vi "总磷总氮测量数据储存.vi"   [LabVIEW 2016, in "斯坦道总氮V2.lvlib"]
uses:
  <vilib>/ptbypt/NI_PtbyPt.lvlib
types:
  T1 = cluster{"跨度值":dbl, "零点标准液浓度":dbl, "跨度标准液浓度":dbl, "标准液标准浓度":dbl}
  T2 = cluster{"系统时间":timestamp, "工作状态":u16, "测量模式":enum16{"待机", "连续模式", "周期模式", "定点模式", "受控模式", "手动模式"}, "告警代码":u16, "故障代码":u16, "日志代码":u16, "软件版本":u16, "F0":sgl, "F1":sgl, "F2":sgl, "F3":sgl, "T":sgl, "H":sgl, "id":u16, "flowid":u16, "量程":u16, "总磷控温温度1":sgl, "营养盐控温温度2":sgl, "ADC":sgl}
  T3 = cluster{"运行模式":enum16{"维护模式", "常规模式", "应急模式", "质控模式", "性能测试"}, "质控频次":enum16{"关闭", "每天", "星期一", "星期二", "星期三", "星期四", "星期五", "星期六", "星期日"}, "空白核查时间":u16, "跨度核查时间":u16, "测量间隔":dbl}
  T4 = cluster{"因子编码":u32, "单位":u16, "标样参考值":sgl, "水样数据时间":timestamp, "水样实测值":sgl, "水样数据标识":string, "标样数据时间":timestamp, "标样实测值":sgl, "标样数据标识":string, "空白数据时间":timestamp, "空白实测值":sgl, "空白数据标识":string, "零点核查数据时间":timestamp, "零点核查实测值":sgl, "零点核查数据标识":string, "跨度核查数据时间":timestamp, "跨度核查实测值":sgl, "跨度核查数据标识":string, "加标回收数据时间":timestamp, "加标回收实测值":sgl, "加标回收数据标识":string, "平行样数据时间":timestamp, "平行样实测值":sgl, "平行样数据标识":string, "F0":sgl, "F1":sgl, "F2":sgl, "F3":sgl, "F4":sgl, "F5":sgl, "F6":sgl, "F7":sgl, "温度":sgl, "湿度":sgl, "X值":sgl, "fidrange":u16}[]
  T5 = cluster{"系统时间":timestamp, "工作状态":u16, "测量模式":enum16{"待机", "连续模式", "周期模式", "定点模式", "受控模式", "手动模式"}, "告警代码":u16, "故障代码":u16, "日志代码":u16, "软件版本":u16, "F0":sgl, "F1":sgl, "F2":sgl, "F3":sgl, "T":sgl, "H":sgl, "id":u16, "flowid":u16, "量程":u16, "总磷控温温度1":sgl, "营养盐控温温度2":sgl, "ADC":sgl}[]
  T6 = cluster{"总磷跨度值":dbl, "总磷零点标准液浓度":dbl, "总磷跨度标准液浓度":dbl, "总磷标准液标准浓度":dbl, "总氮跨度值":dbl, "总氮零点标准液浓度":dbl, "总氮跨度标准液浓度":dbl, "总氮标准液标准浓度":dbl, "氨氮跨度值":dbl, "氨氮零点标准液浓度":dbl, "氨氮跨度标准液浓度":dbl, "氨氮标准液标准浓度":dbl}
  T7 = cluster{"因子编码":u32, "单位":u16, "标样参考值":sgl, "水样数据时间":timestamp, "水样实测值":sgl, "水样数据标识":string, "标样数据时间":timestamp, "标样实测值":sgl, "标样数据标识":string, "空白数据时间":timestamp, "空白实测值":sgl, "空白数据标识":string, "零点核查数据时间":timestamp, "零点核查实测值":sgl, "零点核查数据标识":string, "跨度核查数据时间":timestamp, "跨度核查实测值":sgl, "跨度核查数据标识":string, "加标回收数据时间":timestamp, "加标回收实测值":sgl, "加标回收数据标识":string, "平行样数据时间":timestamp, "平行样实测值":sgl, "平行样数据标识":string, "F0":sgl, "F1":sgl, "F2":sgl, "F3":sgl, "F4":sgl, "F5":sgl, "F6":sgl, "F7":sgl, "温度":sgl, "湿度":sgl, "X值":sgl, "fidrange":u16}
  T8 = cluster{"时间标识":timestamp, "测量模式":enum16{"维护数据", "水样测试", "标样核查", "零点核查", "跨度核查", "空白测试", "平行样测试", "加标回收", "空白校准", "标样校准", "初始化（清洗）", "快捷测试"}, "数据标记表":string, "监测值":sgl, "单位":u16, "数据标识":string, "因子编码":u32, "标样参考值":sgl, "F0":sgl, "F1":sgl, "F2":sgl, "F3":sgl, "F4":sgl, "F5":sgl, "F6":sgl, "F7":sgl, "X":sgl, "温度":sgl, "湿度":sgl, "量程标识":string, "SN":string, "跨度值":sgl, "X1":sgl}
  T9 = typedef "斯坦道总氮V2.lvlib/关键参数.ctl" = cluster{"测量量程":sgl, "测量检出限":sgl, "测量精度":sgl, "测量间隔":sgl, "消解温度":sgl, "消解时长":sgl, "三项式系数":sgl, "二次多项式系数":sgl, "曲线斜率":sgl, "曲线截距":sgl, "线性相关系数":sgl, "空白校准时间":timestamp, "标样校准时间":timestamp, "测量信号值":sgl, "稀释倍数":sgl, "空白标定系数":sgl, "量程系数":sgl}
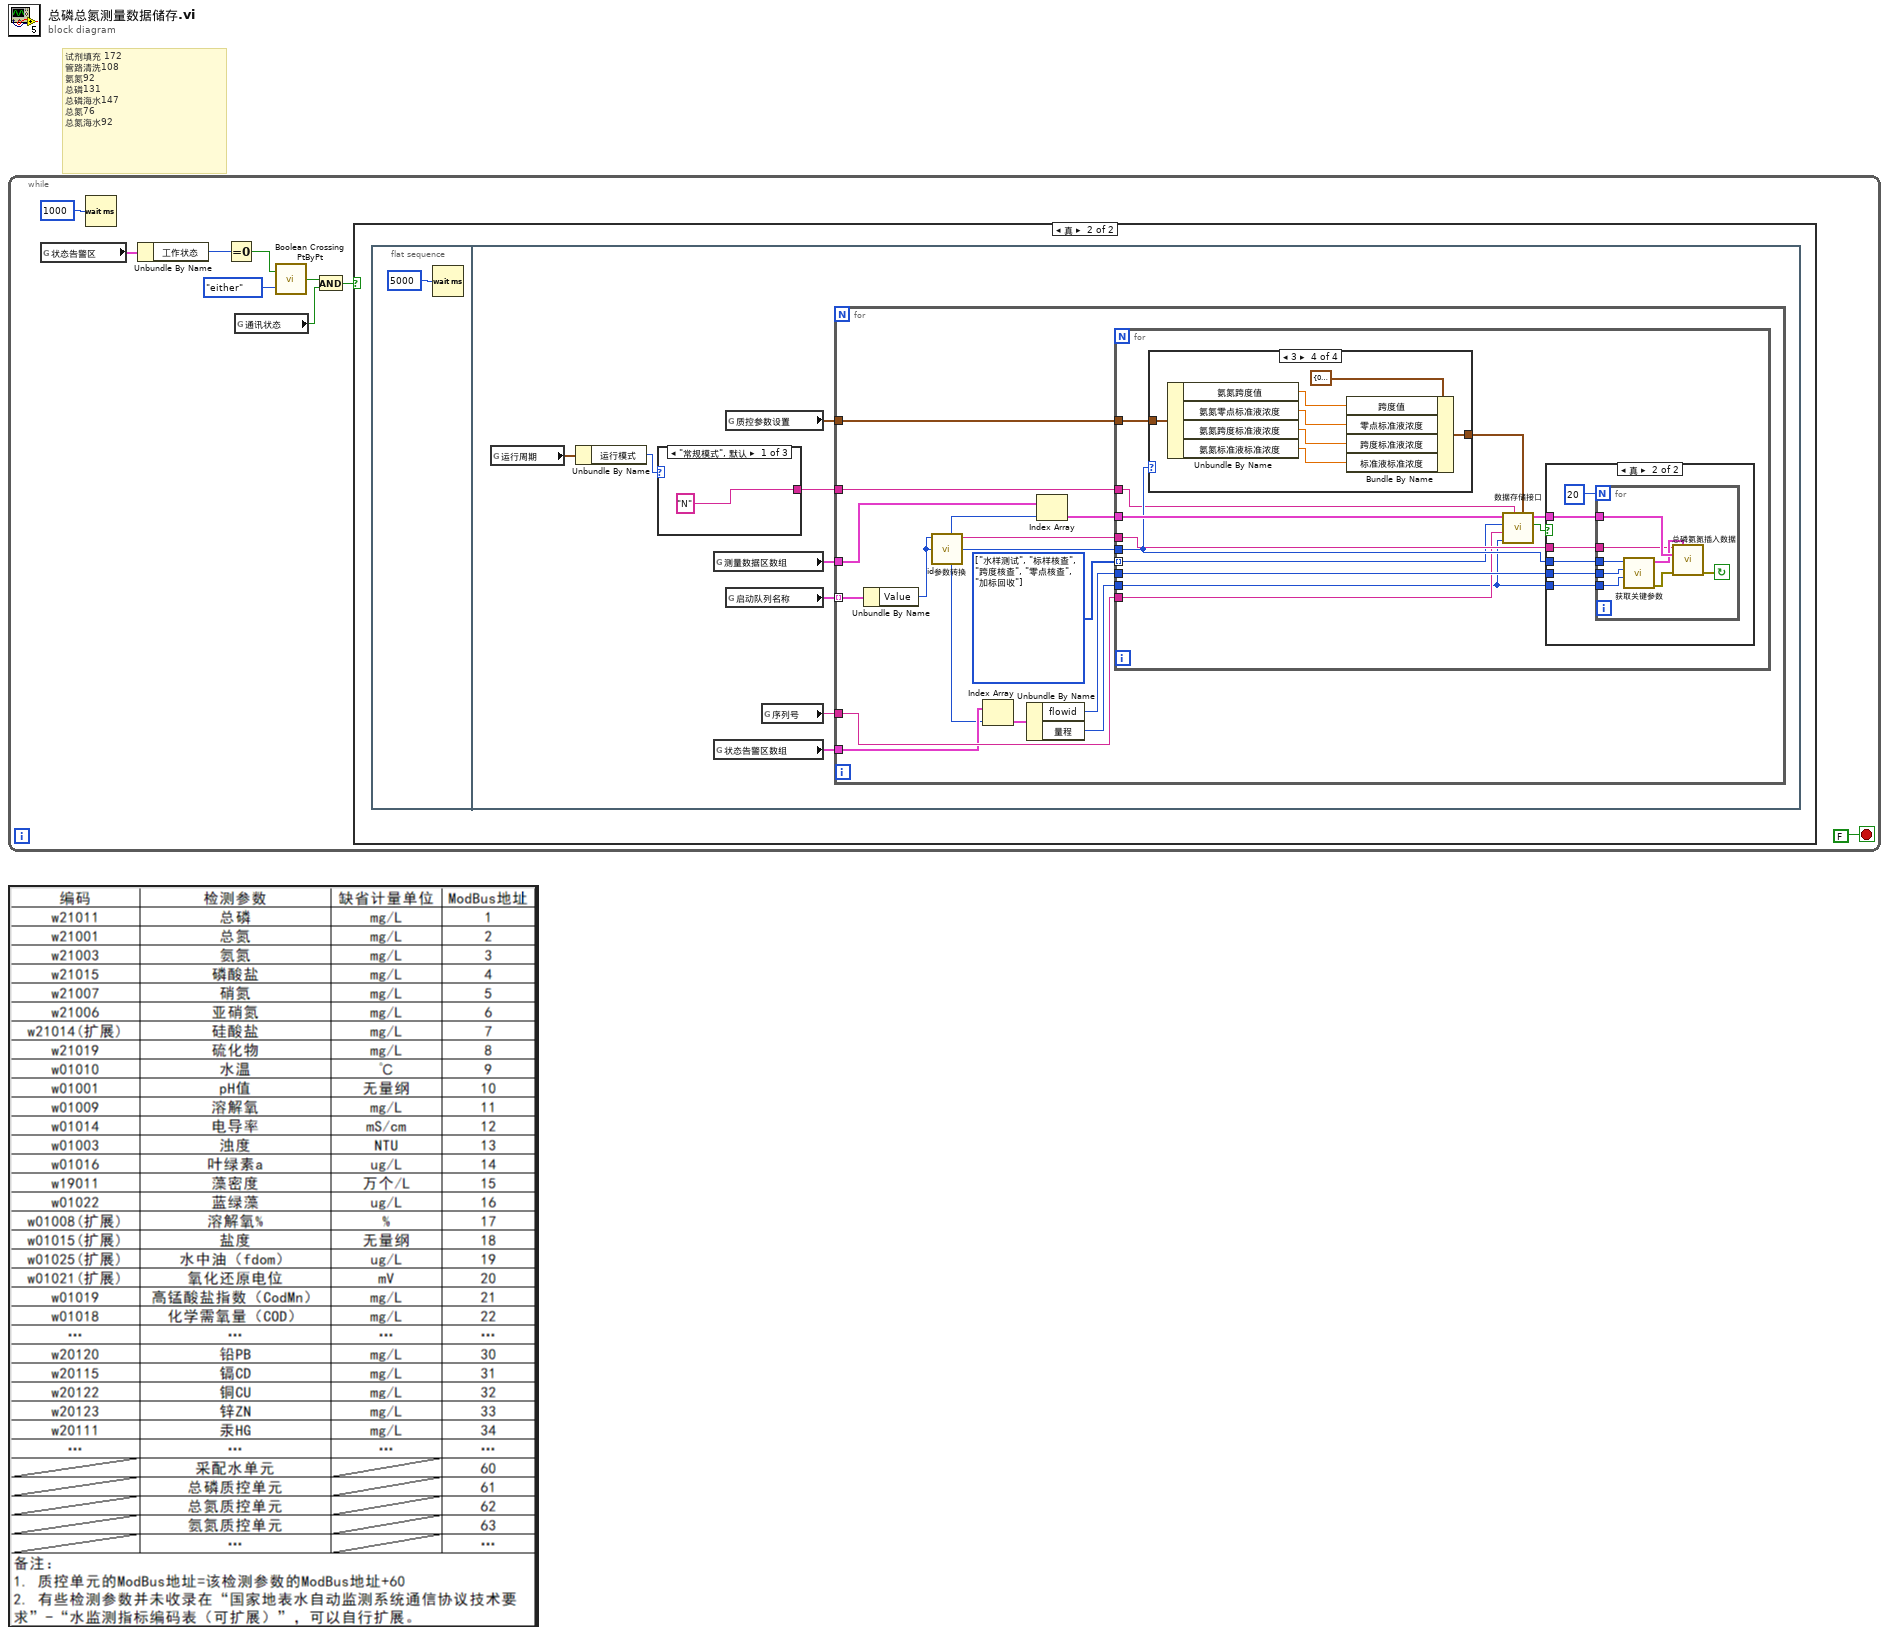
[diagram p0: block diagram]
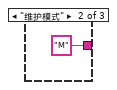
[diagram p3: hidden frame]
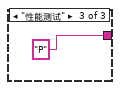
[diagram p4: hidden frame]
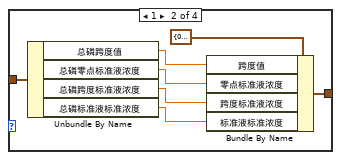
[diagram p7: hidden frame]
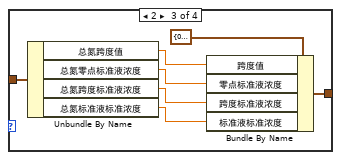
[diagram p8: hidden frame]
diagram:
  # "试剂填充 172 \n管路清洗108\n氨氮92\n总磷131\n总磷海水147\n总氮76\n总氮海水92"
  n1 = while {
    stop <- FALSE stop-if-true
    n2 = global read "VAR总磷总氮全局变量.vi" "状态告警区"() -> (w8:T2)
    n3 = Wait (ms)(milliseconds to wait=u32 1000 ("等待时间（毫秒）")) -> ()  [unwired: 1 out]
    n4 = Unbundle By Name(w8) -> ("工作状态"=w6:u16)
    n5 = Equal To 0?(x=w6) -> (x = 0?=w3:bool)
    n6 = global read "VAR总磷总氮全局变量.vi" "通讯状态"() -> (w1:bool)
    n7 = call <vilib>:"Boolean Crossing PtByPt.vi"("direction"=enum16{"either", "false-true", "true-false"}."either", "input"=w3) -> ("crossing"=w4:bool)  [unwired: 1 in]
    n8 = And(x=w4, y=w1) -> (x .and. y?=w2:bool)
    n9 = case shown="真" w2 {
      frame False {
      }
      frame True {
        n10 = flat-sequence {
          frame #0 {
            n11 = Wait (ms)(milliseconds to wait=u32 5000 ("等待时间（毫秒）")) -> ()  [unwired: 1 out]
          }
          frame #1 {
            n12 = global read "总磷总氮断电保存全局变量.vi" "运行周期"() -> (w14:T3)
            n13 = Unbundle By Name(w14) -> ("运行模式"=w12:enum16{"维护模式", "常规模式", "应急模式", "质控模式", "性能测试"})
            n14 = case shown="\"常规模式\", 默认" w12 {
              tunnel: ["N" "M" "P"] -> w11
              frame "常规模式", Default {
              }
              frame "维护模式" {
              }
              frame "性能测试" {
              }
            }
            n15 = global read "VAR总磷总氮全局变量.vi" "测量数据区数组"() -> (w15:T4)
            n16 = global read "VAR总磷总氮全局变量.vi" "状态告警区数组"() -> (w13:T5)
            n17 = global read "总磷总氮断电保存全局变量.vi" "质控参数设置"() -> (w18:T6)
            n18 = global read "总磷总氮断电保存全局变量.vi" "启动队列名称"() -> (w16:cluster{"String":string, "Value":u16}[])
            n19 = global read "VAR总磷总氮全局变量.vi" "序列号"() -> (w17:string)
            n20 = for {
              tunnel: w18 -> [w35]
              tunnel: w11 -> [w33]
              tunnel: w17 -> [w32]
              tunnel: w16 -> [w31] mode=indexing
              tunnel: w15 -> [w28]
              tunnel: w13 -> [w26]
              w34 = enum16{"水样测试", "标样核查", "跨度核查", "零点核查", "加标回收"}[] [enum."水样测试", enum."标样核查", enum."跨度核查", enum."零点核查", enum."加标回收"] items=["水样测试", "标样核查", "跨度核查", "零点核查", "加标回收"]
              n21 = Unbundle By Name(w31) -> ("Value"=w30:u16)
              n22 = call "id参数转换.vi"("id"=w30) -> ("table输出"=w29:string, "数组资源索引"=w25:i32)  [unwired: 9 in]
              n23 = Index Array(array=w26, index=w25) -> (element=w24:T2)
              n24 = Unbundle By Name(w24) -> ("flowid"=w23:u16, "量程"=w22:u16)
              n25 = Index Array(array=w28, index=w25) -> (element=w27:T7)
              n26 = for {
                tunnel: w35 -> [w46]
                tunnel: w27 -> [w44]
                tunnel: w23 -> [w43]
                tunnel: w22 -> [w37]
                tunnel: w30 -> [w42]
                tunnel: w29 -> [w41]
                tunnel: w34 -> [w40] mode=indexing
                tunnel: w33 -> [w39]
                tunnel: w32 -> [w38]
                n27 = case shown="3" w42 {
                  tunnel: w46 -> [_ w68 w75 w82]
                  tunnel: [_ w66 w73 w80] -> w45
                  frame 0, Default {
                  }
                  frame 1 {
                    n28 = Unbundle By Name(w68) -> ("总磷跨度值"=w65:dbl, "总磷零点标准液浓度"=w64:dbl, "总磷跨度标准液浓度"=w63:dbl, "总磷标准液标准浓度"=w62:dbl)
                    n29 = Bundle By Name(cluster=T1 {"跨度值"=0.0, "零点标准液浓度"=0.0, "跨度标准液浓度"=0.0, "标准液标准浓度"=0.0} ("质控参数设置"), "跨度值"=w65, "零点标准液浓度"=w64, "跨度标准液浓度"=w63, "标准液标准浓度"=w62) -> (w66:T1)
                  }
                  frame 2 {
                    n30 = Unbundle By Name(w75) -> ("总氮跨度值"=w72:dbl, "总氮零点标准液浓度"=w71:dbl, "总氮跨度标准液浓度"=w70:dbl, "总氮标准液标准浓度"=w69:dbl)
                    n31 = Bundle By Name(cluster=T1 {"跨度值"=0.0, "零点标准液浓度"=0.0, "跨度标准液浓度"=0.0, "标准液标准浓度"=0.0} ("质控参数设置"), "跨度值"=w72, "零点标准液浓度"=w71, "跨度标准液浓度"=w70, "标准液标准浓度"=w69) -> (w73:T1)
                  }
                  frame 3 {
                    n32 = Unbundle By Name(w82) -> ("氨氮跨度值"=w79:dbl, "氨氮零点标准液浓度"=w78:dbl, "氨氮跨度标准液浓度"=w77:dbl, "氨氮标准液标准浓度"=w76:dbl)
                    n33 = Bundle By Name(cluster=T1 {"跨度值"=0.0, "零点标准液浓度"=0.0, "跨度标准液浓度"=0.0, "标准液标准浓度"=0.0} ("质控参数设置"), "跨度值"=w79, "零点标准液浓度"=w78, "跨度标准液浓度"=w77, "标准液标准浓度"=w76) -> (w80:T1)
                  }
                }
                n34 = call "数据存储接口.vi"("质控参数设置"=w45, "数据标记表"=w39, "量程"=w37, "SN"=w38, "数据存储模式"=w40, "测量数据区"=w44) -> ("x >= y?"=w36:bool, "data输出"=w47:T8)  [unwired: 4 in]
                n35 = case shown="真" w36 {
                  tunnel: w47 -> [_ w53]
                  tunnel: w43 -> [_ w52]
                  tunnel: w42 -> [_ w51]
                  tunnel: w41 -> [_ w50]
                  tunnel: w37 -> [_ w49]
                  frame False {
                  }
                  frame True {
                    n36 = for {
                      N: 20 -> [_]
                      tunnel: w53 -> [w61]
                      tunnel: w52 -> [w58]
                      tunnel: w51 -> [w57]
                      tunnel: w50 -> [w56]
                      tunnel: w49 -> [w55]
                      stop <- w54 continue-if-true
                      n37 = call "获取关键参数.vi"("量程"=w55, "flowid"=w58, "id"=w57) -> ("error out"=w60:errorcluster, "关键参数"=w59:T9)  [unwired: 7 in]
                      n38 = call "总磷氨氮插入数据.vi"("table"=w56, "关键参数"=w59, "data"=w61, "error in (no error)"=w60) -> ("error out"=w54:errorcluster)  [unwired: 11 in]
                    }
                  }
                }
              }
            }
          }
        }
      }
    }
  }
